vi "Process.vi"(8 "error in (no error)":errorcluster, 10 "gate":T1, 11 "process index":i32) -> (0 "error out":errorcluster)   [LabVIEW 2015]
doc: "Checks the gate and blinks the indicator."
uses:
  Gates/Source/Gate.ctl
  Wait.vi
  Stop.vi
  Gates/Gates.lvlib
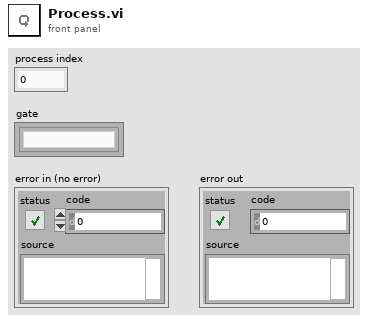
[diagram p1: front panel]
types:
  T1 = typedef "Gates.lvlib/Gate.ctl" = refnum<k1>
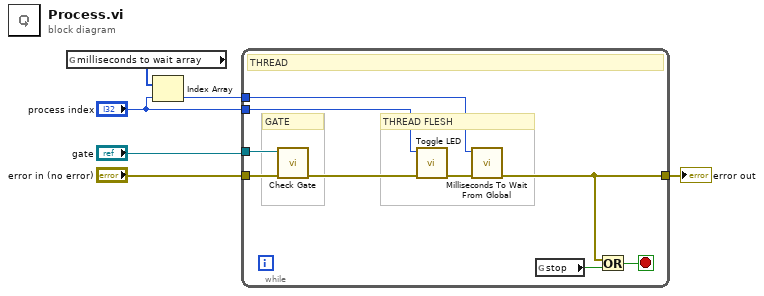
[diagram p0: block diagram]
diagram:
  n1 = global read "Wait.vi" "milliseconds to wait array"() -> (w3:u32[])
  n2 = Index Array(array=w3, index="process index") -> (element=w2:u32)
  n3 = while {
    tunnel: "process index" -> [w15]
    tunnel: "error in (no error)" -> [w10]
    tunnel: [w7] -> w6
    tunnel: "gate" -> [w11]
    tunnel: w2 -> [w9]
    stop <- w13 stop-if-true
    # "GATE"
    # "THREAD FLESH"
    # "THREAD"
    n4 = call "Check Gate.vi"("error in (no error)"=w10, "gate"=w11) -> ("error out"=w12:errorcluster)  [unwired: 7 in, 2 out]
    n5 = call "Toggle LED.vi"("error in (no error)"=w12, "process index"=w15) -> ("error out"=w8:errorcluster)  [unwired: 8 in, 1 out]
    n6 = call "Milliseconds To Wait From Global.vi"("error in (no error)"=w8, "milliseconds to wait"=w9) -> ("error out"=w7:errorcluster)  [unwired: 9 in]
    n7 = global read "Stop.vi" "stop"() -> (w14:bool)
    n8 = Or(x=w7, y=w14) -> (x .or. y?=w13:bool)
  }
  "error out" <- w6
